vi "Block_Control_global.vi"() -> ()   [LabVIEW 2010]
panel:
  in  "No of Blocks to PP":i32=1 min=1
  in  "Start Block Number":i32=1 min=1
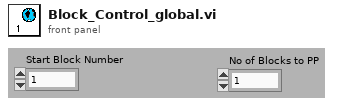
[diagram p1: front panel]
diagram:
